vi "Stop Aquisition.vi"(8 "error in (no error)":errorcluster, 11 "DAQ Controller in":refnum<class "DAQ Controller.lvclass">) -> (0 "error out":errorcluster, 3 "DAQ Controller out":refnum<class "DAQ Controller.lvclass">)   [LabVIEW 2022 SP3, in "DAQ Controller.lvclass"]
uses:
  DAQ Controller.lvclass
  DAQ Controller.lvclass/DAQ Controller.ctl
  XY Stage/Process Actor/Process Framework/Process State Data/Process State Data.lvclass/Process State Data.ctl
  XY Stage/Process Actor/Process Framework/Interlock Q Class/Interlock Q Class.lvclass/Interlock Q Class.ctl
  <vilib>/ActorFramework/Message Enqueuer/Message Enqueuer.lvclass/Message Enqueuer.ctl
  XY Stage/Process Actor/Process Framework/Process State Data/Accessor/Write Abort.vi
  <vilib>/ActorFramework/Message Enqueuer/Enqueue.vi
  DAQ Actor/DAQ Process Messages/Stop Aquisition Msg/Stop Aquisition Msg.lvclass
  C:/Program Files/National Instruments/LabVIEW 2022/vi.lib/ActorFramework/Message/Message.lvclass
  <vilib>/ActorFramework/Message Priority Queue/Priority Enqueue.vi
  <vilib>/ActorFramework/Message Enqueuer/Message Enqueuer.lvclass
  XY Stage/Process Actor/Process Framework/Interlock Q Class/Interlock Q Class.lvclass
  XY Stage/Process Actor/Process Framework/Process State Data/Process State Data.lvclass
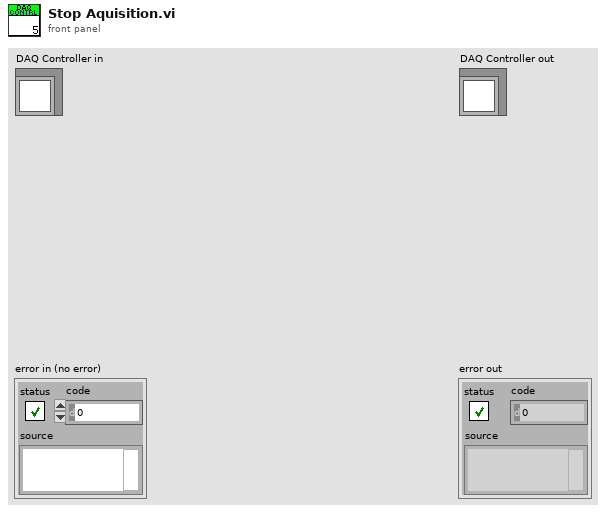
[diagram p1: front panel]
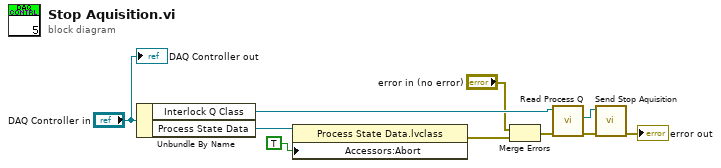
[diagram p0: block diagram]
diagram:
  n1 = Unbundle By Name("DAQ Controller in") -> ("Interlock Q Class"=w9:refnum<class "Interlock Q Class.lvclass">, "Process State Data"=w3:refnum<data-value>)
  n2 = property class="Process State Data.lvclass"(reference=w3, "Accessors:Abort"=TRUE ("Abort")) -> (error out=w1:errorcluster)  [unwired: 1 in, 1 out]
  n3 = Merge Errors("error in (no error)", w1) -> (w2:errorcluster)
  n4 = call "Read Process Q.vi"("error in (no error)"=w2, "Interlock Q Class in"=w9) -> ("error out"=w5:errorcluster, "Actor Framework:Message Enqueuer"=w8:refnum<class "Message Enqueuer.lvclass">)  [unwired: 7 in, 1 out]
  n5 = call "Send Stop Aquisition.vi"("error in (no error)"=w5, "Message Enqueuer"=w8) -> ("error out"=→"error out":errorcluster)  [unwired: 8 in, 1 out]
  "DAQ Controller out" <- "DAQ Controller in"
